vi "DCS.vi"(3 "error in":errorcluster) -> (10 "error out":errorcluster)   [LabVIEW 2013]
uses:
  <vilib>/Utility/miscctls.llb/LVPointTypeDef.ctl
  <vilib>/gmath/NumericalOptimization/Nonlinear Curve Fit LM.vi
  <userlib>/Accelerator/User Interface/Controls/dcs points.ctl
  <userlib>/Accelerator/User Interface/Controls/dcs_spot.ctl
  <vilib>/gmath/NI_Gmath.lvlib
panel:
  in  "Points to Check Noise":i32=2000
  in  "Color bar Control":cluster{dbl, u32}[](array[cluster])
  in  "stop":bool
  in  "Tab Control":T1(tab)
  out "Intensity Graph":dbl[][](graph)
  in  "Spot Save Folder":path=path "C:/Users/Clavius/Desktop/Spot Images"
  in  "Save Spot Image":bool
  in  "Clear Spot/Track":bool
  in  "Particle Limit":i64=500 min=0 step=10
  out "Laser spot\nMove (mm)":dbl[](array[numeric])=[nan, nan] format="%#.3g"
  out "Avg. Freq. (Hz)":dbl
  in  "Orange Cursor Position":dbl[](array[numeric])=[0.0, 0.0] min=-12.0 max=12.0 step=0.1 format="%.3g"
  out "Spot Widths":dbl[](array[numeric]) format="%.6g"
  out "Countdown to\nnext track point":i32=1
  out "XY Graph":cluster{"Y":dbl[], "Y":dbl[]}[](graph)
  in  "Load old position\nto Orange Cursor":bool
  in  "Set Orange Cursor\nto current position":bool
  out "# of Particles\nin Spot":dbl
  out "Current Spot Pos":dbl[](array[numeric])=[nan, nan] format="%.3g"
  in  "# of shots to calculate spot":i32=20
  out "Spot Size over time":dbl[][](graph)
  out "Filtered Signals":dbl[][](graph)
  out "Unfiltered Signals":ext[][](graph)
  in  "Auto Threshold":bool
  out "Sampling Frequency":u16(ring) items=["40 MHz", "20 MHz", "10 MHz", "5 MHz", "2.5 MHz", "1 MHz", "100 kHz", "10 kHz"]
  out "Length of Sample":dbl caption="s" format="%^#_3g"
  out "Memory Address Pointer":ext
  out "Post trigger Size":ext
  out "Pretrigger Size":ext
  out "Trigger Generation register":i32=23 format="%.0b"
  out "status register":i8=4 format="%08b"
  out "control register":i16=23 format="%015b"
  in  "Posttrigger size":i32
  in  "Acquisition Rate":u16(ring) items=["40 MHz", "20 MHz", "10 MHz", "5 MHz", "2.5 MHz", "1 MHz", "100 kHz", "10 kHz"]
  in  "Pretrigger size":i32=1000
  in  "Rising or falling?":bool
  out "Running Errors":errorcluster
  in  "Jorger TR slot":i32=3
  in  "Channels":i32[](array[numeric])=[0, 1, 2, 3, 4, 5, 6, 7]
  in  "Median Filter Rank":i32=30
  in  "Thresholds":ext[](array[numeric])
  in  "Level Buffer":i32=25
  in  "y":bool
  out "output":i32
  # "DAQ Parameter Indicators"
  # "DAQ Parameter Controls"
  # "Falling"
  # "Rising"
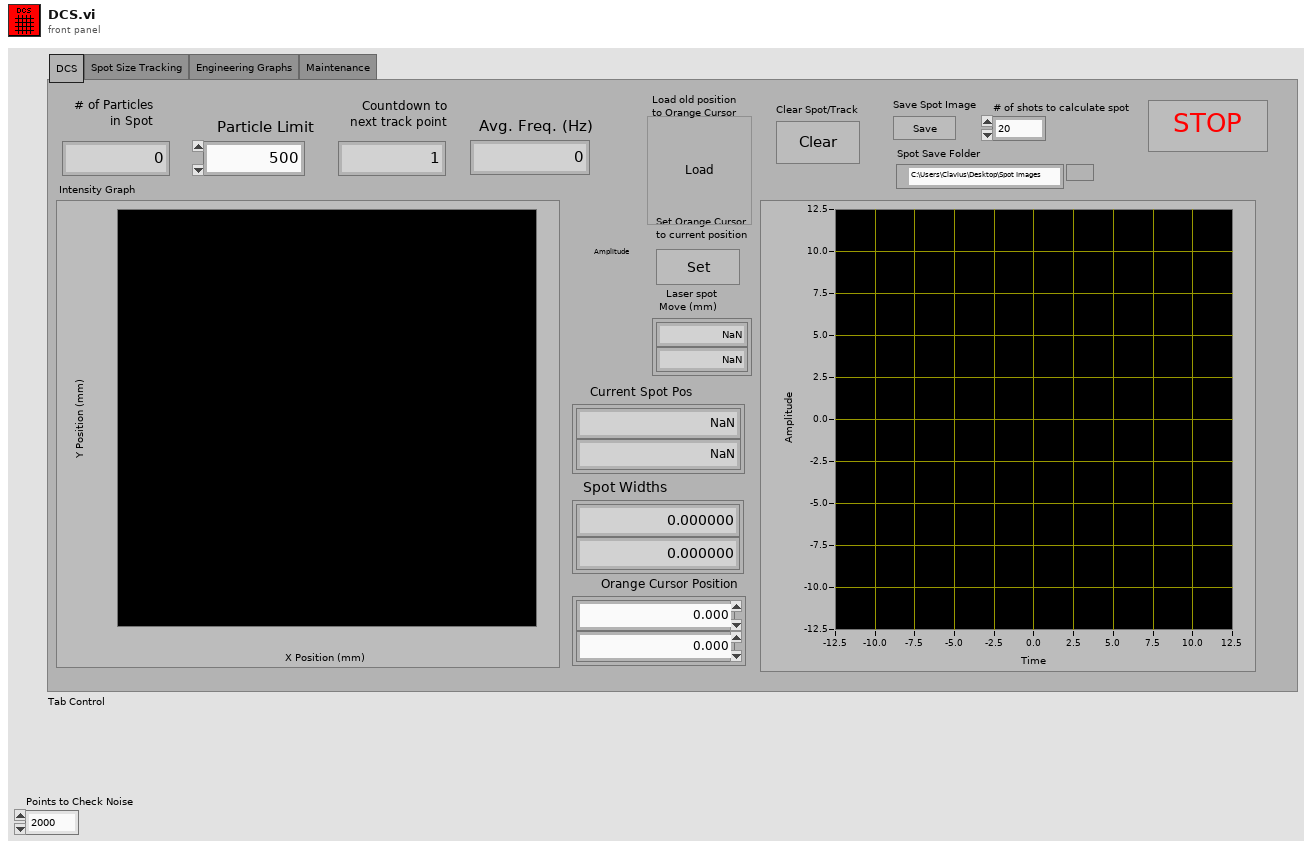
[diagram p1: front panel]
types:
  T1 = enum32{"DCS", "Spot Size Tracking", "Engineering Graphs", "Maintenance"}
  T2 = typedef "LVPointTypeDef.ctl" = cluster{"Horizontal":i16, "Vertical":i16}
  T3 = typedef "dcs_spot.ctl" = cluster{"DCS spot ID":i32, "Integer Timestamp":i64, "Spot X":dbl, "Spot Y":dbl, "Spot Width X":dbl, "Spot Width Y":dbl, "Spot Size":i32, "Experiment Settings ID":i32}
  T4 = typedef "dcs points.ctl" = cluster{"Integer Timestamp":i64, "X":dbl, "Y":dbl, "DCS spot ID":i32}
  T5 = typedef "imagedata.ctl" = cluster{"image type":i32, "image depth":i32, "image":u8[], "mask":u8[], "colors":u32[], "Rectangle":cluster{"left":i16, "top":i16, "right":i16, "bottom":i16}}
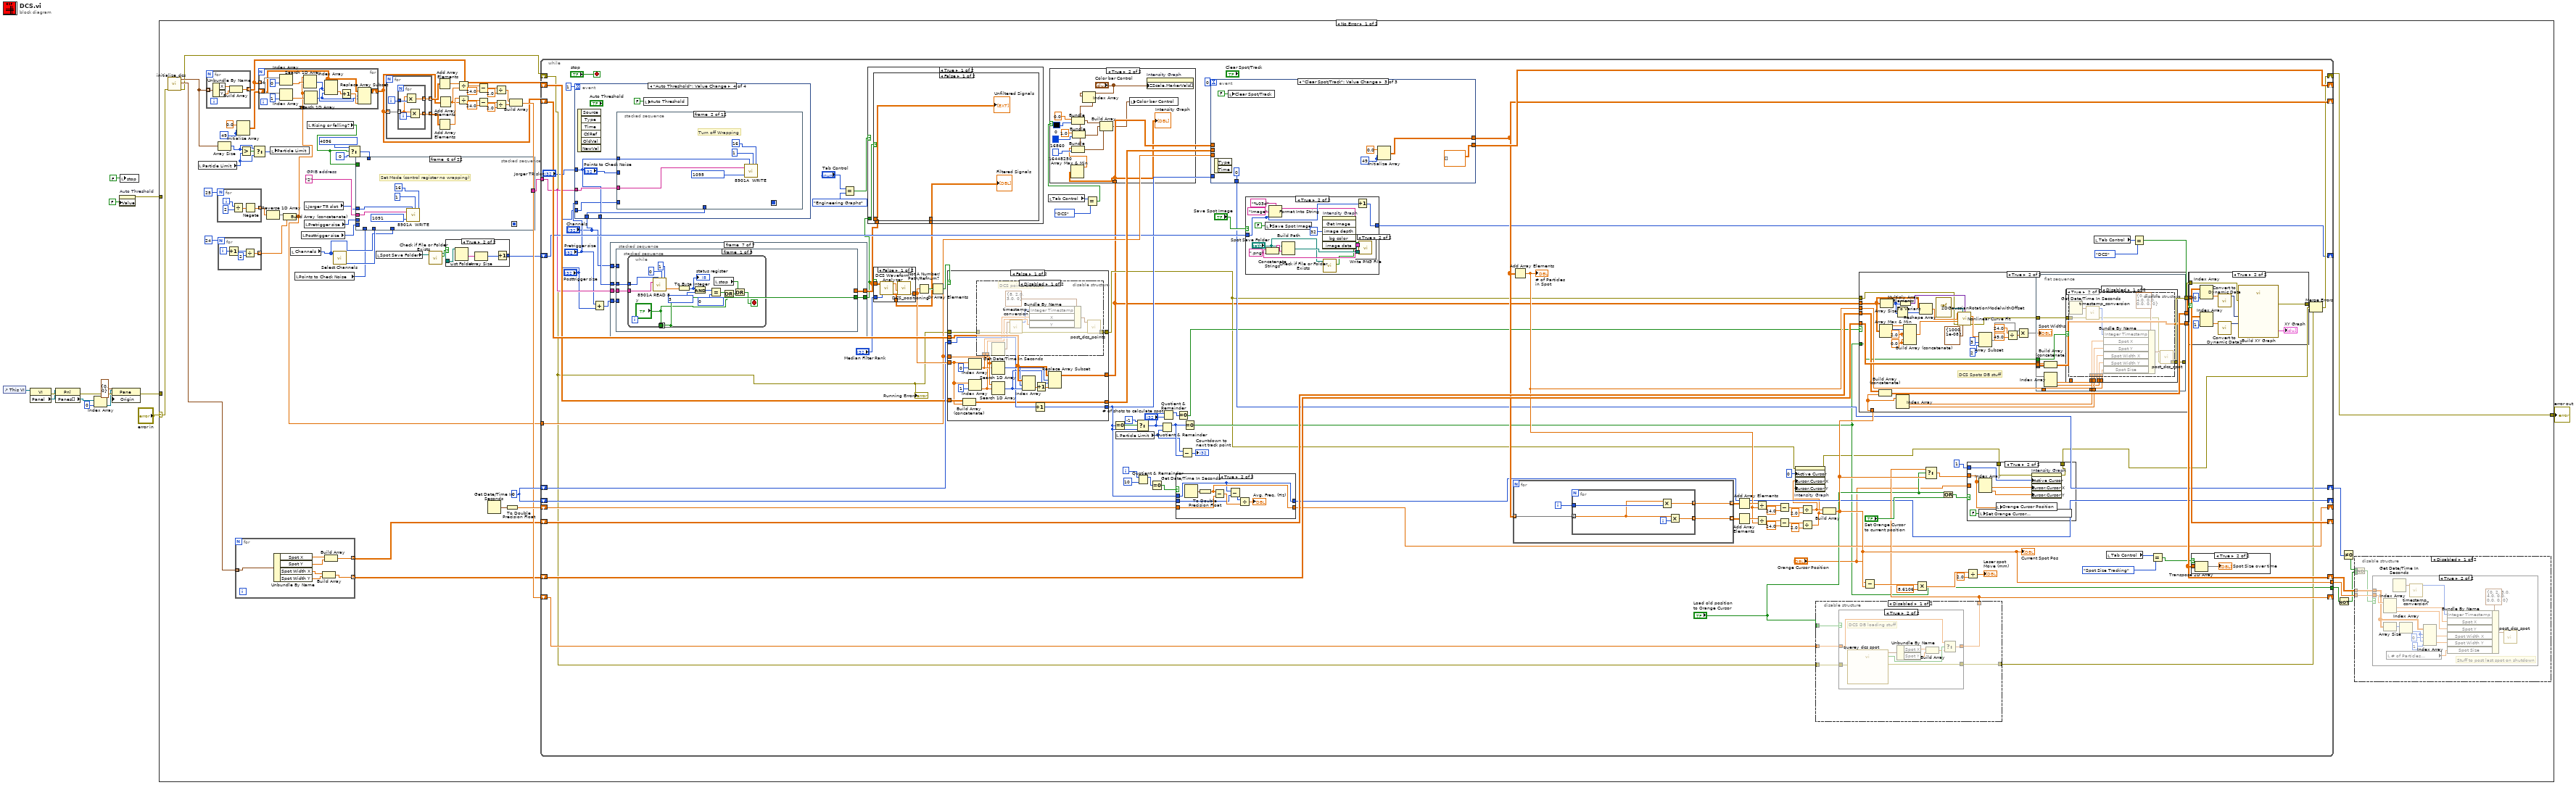
[diagram p0: block diagram]
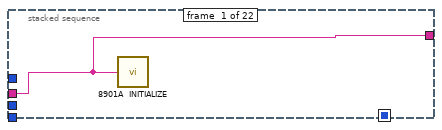
[diagram p4: hidden frame]
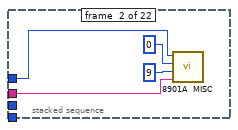
[diagram p5: hidden frame]
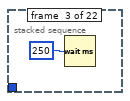
[diagram p6: hidden frame]
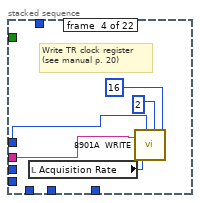
[diagram p7: hidden frame]
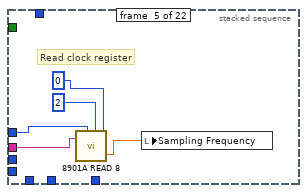
[diagram p8: hidden frame]
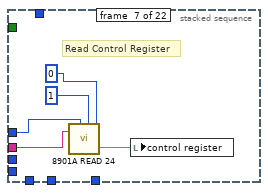
[diagram p9: hidden frame]
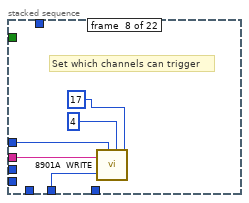
[diagram p10: hidden frame]
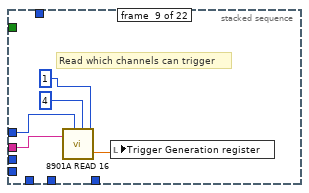
[diagram p11: hidden frame]
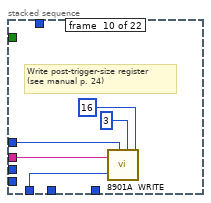
[diagram p12: hidden frame]
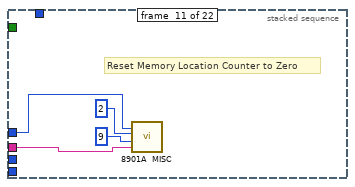
[diagram p13: hidden frame]
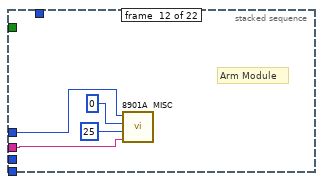
[diagram p14: hidden frame]
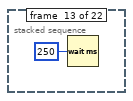
[diagram p15: hidden frame]
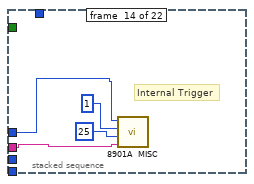
[diagram p16: hidden frame]
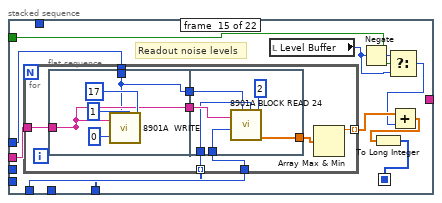
[diagram p17: hidden frame]
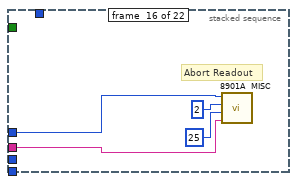
[diagram p18: hidden frame]
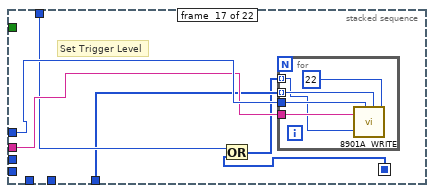
[diagram p19: hidden frame]
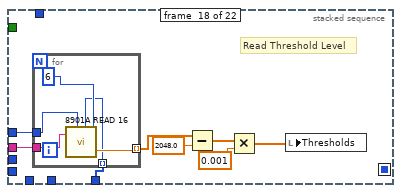
[diagram p20: hidden frame]
diagram:
  n1 = control-ref of="This VI"() -> (w11:refnum<vi>)
  n2 = property class="VI"(reference=w11) -> (error out=w10:errorcluster, "Panel"=w9:refnum<vi>)  [unwired: 1 in, 1 out]
  n3 = property class="Pnl"(reference=w9, error in=w10) -> (error out=w8:errorcluster, "Panes[]"=w7:refnum<vi>[])  [unwired: 1 out]
  n4 = Index Array(array=w7, index=0) -> (element=w5:refnum<vi>)
  n5 = property class="Pane"(reference=w5, error in=w8, "Origin"=T2 {"Horizontal"=0, "Vertical"=0}) -> (error out=w3:errorcluster)  [unwired: 1 out]
  n6 = property on="Auto Threshold" class="Bool (strict)"("Value"=FALSE ("Auto Threshold")) -> (error out=w1:errorcluster)  [unwired: 2 in, 1 out]
  n7 = local write "stop"(FALSE ("stop")) -> ()
  n8 = case shown="No Error" "error in" {
    selector: "error in" -> [w33 w956]
    tunnel: [w32 w956] -> w13
    tunnel: w3 -> [_ _]
    tunnel: w1 -> [_ _]
    frame No Error {
      w26 = "2"  # GPIB address
      w52 = 49 ("dimension size")
      w55 = 0
      n9 = call <userlib>:"initialize_dcs.vi"("error in (no error)"=w33) -> ("error out"=w27:errorcluster, "Dust Spot Array"=w44:T3[], "Dust Point Array"=w38:T4[])  [unwired: 8 in]
      n10 = local read "Particle Limit"() -> (w35:i64)
      n11 = for {
        tunnel: [w255] -> w43 mode=indexing
        tunnel: w38 -> [w254] mode=indexing
        n12 = Unbundle By Name(w254) -> ("X"=w257:dbl, "Y"=w256:dbl)
        n13 = Build Array(w257, w256) -> (w255:dbl[])
      }
      n14 = for {
        N: 25 -> [_]
        tunnel: [w271] -> w75 mode=indexing
        i -> [w274]
        n15 = Divide(x=w274, y=2) -> (x/y=w272:dbl)
        n16 = Negate(x=w272) -> (-x=w271:dbl)
      }
      n17 = Array Size(array=w38) -> (size(s)=w36:i32)
      n18 = for {
        N: 24 -> [_]
        tunnel: [w268] -> w73 mode=indexing
        i -> [w270]
        n19 = Increment(x=w270) -> (x+1=w267:i32)
        n20 = Divide(x=w267, y=2) -> (x/y=w268:dbl)
      }
      n21 = for {
        tunnel: [w249] -> w47 mode=indexing
        tunnel: [w248] -> w48 mode=indexing
        tunnel: w44 -> [w247] mode=indexing
        n22 = Unbundle By Name(w247) -> ("Spot X"=w253:dbl, "Spot Y"=w252:dbl, "Spot Width X"=w251:dbl, "Spot Width Y"=w250:dbl)
        n23 = Build Array(w251, w250) -> (w249:dbl[])
        n24 = Build Array(w253, w252) -> (w248:dbl[])
      }
      n25 = Initialize Array(0.0 ("element"), w52, w52) -> (w51:dbl[][])
      n26 = Greater?(x=w36, y=w35) -> (0:w37:bool)
      n27 = Select(t=w36, s=w37, f=w35) -> (s? t:f=w34:i64)
      n28 = Reverse 1D Array(array=w75) -> (reversed array=w74:dbl[])
      n29 = local write "Particle Limit"(w34) -> ()
      n30 = Build Array (concatenate)(w74, w73) -> (w49:dbl[])
      n31 = for {
        tunnel: w43 -> [w244] mode=indexing
        tunnel: w49 -> [w235]
        shift-right: [w236] -> w42
        shift-left: w51 -> [w237]
        n32 = Index Array(array=w244, index=0) -> (element=w243:dbl)
        n33 = Index Array(array=w244, index=1) -> (element=w242:dbl)
        n34 = Search 1D Array(1D array=w235, element=w243) -> (index of element=w239:i32)  [unwired: 1 in]
        n35 = Search 1D Array(1D array=w235, element=w242) -> (index of element=w238:i32)  [unwired: 1 in]
        n36 = Index Array(array=w237, index (row)=w239, index (col)=w238) -> (element=w241:dbl)
        n37 = Increment(x=w241) -> (x+1=w240:dbl)
        n38 = Replace Array Subset(array=w237, new element=w240, index (row)=w239, index (col)=w238) -> (w236:dbl[][])
      }
      n39 = local read "Channels"() -> (w17:i32[])
      n40 = local read "Points to Check Noise"() -> (w16:i32)
      n41 = local read "Posttrigger size"() -> (w22:i32)
      n42 = local read "Jorger TR slot"() -> (w24:i32)
      n43 = local read "Pretrigger size"() -> (w23:i32)
      n44 = local read "Rising or falling?"() -> (w15:bool)
      n45 = call <userlib>:"Select Channels.vi"("Channels"=w17) -> ("Channels in Use"=w21:u32)  [unwired: 10 in]
      n46 = Select(t=4096, s=w15, f=0) -> (s? t:f=w18:i32)
      n47 = stacked-sequence {
        seq-local: [_ _ _ _ _ _ _ _ _ _ _ _ _ _ w156 _ _ _ _ _ _ _] -> [_ _ _ _ _ _ _ _ _ _ _ _ _ _ _ _ w186 _ _ _ _ _]
        tunnel: w24 -> [_ w99 _ w106 w111 w114 w121 w125 w130 w136 w140 w143 _ w148 w158 w183 w191 w204 w212 w217 w222 w227]
        tunnel: w26 -> [w98 w100 _ w105 w110 w115 w120 w126 w131 w135 w139 w144 _ w149 w162 w182 w190 w203 w211 w216 w221 w226]
        tunnel: w23 -> [_ _ _ _ _ _ _ _ _ _ _ _ _ _ _ _ _ _ _ _ w220 _]
        tunnel: w22 -> [_ _ _ _ _ _ _ _ _ _ _ _ _ _ _ _ _ _ w210 _ _ _]
        tunnel: [w98 _ _ _ _ _ _ _ _ _ _ _ _ _ _ _ _ _ _ _ _ _] -> w25
        tunnel: w21 -> [_ _ _ _ _ _ _ w124 _ _ _ _ _ _ _ _ _ _ _ _ _ _]
        tunnel: w16 -> [_ _ _ _ _ _ _ _ _ w134 _ _ _ _ w161 _ _ _ _ _ _ _]
        tunnel: w18 -> [_ _ _ _ _ _ _ _ _ _ _ _ _ _ _ _ w189 _ _ _ _ _]
        tunnel: w17 -> [_ _ _ _ _ _ _ _ _ _ _ _ _ _ w159 _ w188 w198 _ _ _ _]
        tunnel: w15 -> [_ _ _ _ _ _ _ _ _ _ _ _ _ _ w153 _ _ _ _ _ _ _]
        frame #0 {
          n48 = call <instrlib>:"8901A  INITIALIZE.vi"("GPIB address"=w98) -> ()
        }
        frame #1 {
          n49 = call <instrlib>:"8901A  MISC.vi"("GPIB address"=w100, "f"=9, "a"=0, "n"=w99) -> ()
        }
        frame #2 {
          n50 = Wait (ms)(milliseconds to wait=250) -> ()  [unwired: 1 out]
        }
        frame #3 {
          # "Write TR clock register\n(see manual p. 20)"
          n51 = local read "Acquisition Rate"() -> (w104:u16)
          n52 = call <instrlib>:"8901A  WRITE.vi"("data"=w104, "GPIB address"=w105, "n"=w106, "a"=2, "f"=16) -> ()  [unwired: 1 in]
        }
        frame #4 {
          # "Read clock register"
          n53 = call <instrlib>:"8901A READ 8.vi"("GPIB address"=w110, "n"=w111, "a"=2, "f"=0) -> ("output"=w109:ext)  [unwired: 3 in]
          n54 = local write "Sampling Frequency"(w109) -> ()
        }
        frame #5 {
          # "Set Mode (control register no wrapping)"
          n55 = call <instrlib>:"8901A  WRITE.vi"("data"=1091, "GPIB address"=w115, "n"=w114, "a"=1, "f"=16) -> ()  [unwired: 1 in]
        }
        frame #6 {
          # "Read Control Register"
          n56 = call <instrlib>:"8901A READ 24.vi"("GPIB address"=w120, "n"=w121, "a"=1, "f"=0) -> ("output"=w119:ext)  [unwired: 3 in]
          n57 = local write "control register"(w119) -> ()
        }
        frame #7 {
          # "Set which channels can trigger"
          n58 = call <instrlib>:"8901A  WRITE.vi"("data"=w124, "GPIB address"=w126, "n"=w125, "a"=4, "f"=17) -> ()  [unwired: 1 in]
        }
        frame #8 {
          # "Read which channels can trigger"
          n59 = call <instrlib>:"8901A READ 16.vi"("GPIB address"=w131, "n"=w130, "a"=u8 4, "f"=u8 1) -> ("output"=w129:ext)  [unwired: 3 in]
          n60 = local write "Trigger Generation register"(w129) -> ()
        }
        frame #9 {
          # "Write post-trigger-size register\n(see manual p. 24)"
          n61 = call <instrlib>:"8901A  WRITE.vi"("data"=w134, "GPIB address"=w135, "n"=w136, "a"=3, "f"=16) -> ()  [unwired: 1 in]
        }
        frame #10 {
          # "Reset Memory Location Counter to Zero"
          n62 = call <instrlib>:"8901A  MISC.vi"("GPIB address"=w139, "f"=u8 9, "a"=u8 2, "n"=w140) -> ()
        }
        frame #11 {
          # "Arm Module"
          n63 = call <instrlib>:"8901A  MISC.vi"("GPIB address"=w144, "f"=25, "a"=0, "n"=w143) -> ()
        }
        frame #12 {
          n64 = Wait (ms)(milliseconds to wait=u32 250) -> ()  [unwired: 1 out]
        }
        frame #13 {
          # "Internal Trigger"
          n65 = call <instrlib>:"8901A  MISC.vi"("GPIB address"=w149, "f"=u8 25, "a"=u8 1, "n"=w148) -> ()
        }
        frame #14 {
          # "Readout noise levels"
          n66 = for {
            tunnel: w162 -> [w169]
            tunnel: w161 -> [w168]
            tunnel: [w166] -> w160 mode=indexing
            tunnel: w159 -> [w165] mode=indexing
            tunnel: w158 -> [w164]
            n67 = flat-sequence {
              tunnel: [w173] -> _
              tunnel: [w173] -> w170
              tunnel: w169 -> [w173]
              tunnel: w164 -> [w171]
              tunnel: [w171] -> w163
              tunnel: w170 -> [w180]
              tunnel: [w179] -> w167
              tunnel: w168 -> [w178]
              tunnel: w165 -> [w177]
              tunnel: w163 -> [w176]
              frame #0 {
                n68 = call <instrlib>:"8901A  WRITE.vi"("data"=0, "GPIB address"=w173, "n"=w171, "a"=1, "f"=17) -> ()  [unwired: 1 in]
              }
              frame #1 {
                n69 = call <instrlib>:"8901A BLOCK READ 24.vi"("f"=2, "a"=w177, "n"=w176, "GPIB address"=w180, "# points to read"=w178) -> ("output"=w179:ext[])  [unwired: 4 in]
              }
            }
            n70 = Array Max & Min(array=w167) -> (max value=w166:ext)  [unwired: 3 out]
          }
          n71 = local read "Level Buffer"() -> (w155:i32)
          n72 = Negate(x=w155) -> (-x=w154:i32)
          n73 = Select(t=w154, s=w153, f=w155) -> (s? t:f=w152:i32)
          n74 = Add(x=w160, y=w152) -> (x+y=w157:ext[])
          n75 = To Long Integer(number=w157) -> (32bit integer=w156:i32[])
        }
        frame #15 {
          # "Abort Readout"
          n76 = call <instrlib>:"8901A  MISC.vi"("GPIB address"=w182, "f"=25, "a"=2, "n"=w183) -> ()
        }
        frame #16 {
          # "Set Trigger Level"
          n77 = Or(x=w189, y=w186) -> (x .or. y?=w187:i32[])
          n78 = for {
            tunnel: w191 -> [w195]
            tunnel: w190 -> [w194]
            tunnel: w188 -> [w193] mode=indexing
            tunnel: w187 -> [w192] mode=indexing
            n79 = call <instrlib>:"8901A  WRITE.vi"("data"=w192, "GPIB address"=w194, "n"=w195, "a"=w193, "f"=u8 22) -> ()  [unwired: 1 in]
          }
        }
        frame #17 {
          # "Read Threshold Level"
          n80 = for {
            tunnel: w204 -> [w208]
            tunnel: w203 -> [w207]
            tunnel: [w206] -> w201 mode=indexing
            tunnel: w198 -> [w205] mode=indexing
            n81 = call <instrlib>:"8901A READ 16.vi"("GPIB address"=w207, "n"=w208, "a"=w205, "f"=u8 6) -> ("output"=w206:ext)  [unwired: 3 in]
          }
          n82 = Subtract(x=w201, y=2048.0) -> (x-y=w199:ext[])
          n83 = Multiply(x=w199, y=0.001) -> (x*y=w197:ext[])
          n84 = local write "Thresholds"(w197) -> ()
        }
        frame #18 {
          # "Write post-trigger-size register\n(see manual p. 24)"
          n85 = call <instrlib>:"8901A  WRITE.vi"("data"=w210, "GPIB address"=w211, "n"=w212, "a"=3, "f"=16) -> ()  [unwired: 1 in]
        }
        frame #19 {
          # "Read Post trigger size"
          n86 = call <instrlib>:"8901A READ 24.vi"("GPIB address"=w216, "n"=w217, "a"=3, "f"=0) -> ("output"=w215:ext)  [unwired: 3 in]
          n87 = local write "Post trigger Size"(w215) -> ()
        }
        frame #20 {
          # "Write Pretrigger size"
          n88 = call <instrlib>:"8901A  WRITE.vi"("data"=w220, "GPIB address"=w221, "n"=w222, "a"=4, "f"=16) -> ()  [unwired: 1 in]
        }
        frame #21 {
          # "Read Pretrigger size"
          n89 = call <instrlib>:"8901A READ 16.vi"("GPIB address"=w226, "n"=w227, "a"=u8 4, "f"=u8 0) -> ("output"=w225:ext)  [unwired: 3 in]
          n90 = local write "Pretrigger Size"(w225) -> ()
        }
      }
      n91 = local read "Spot Save Folder"() -> (w30:path)
      n92 = for {
        tunnel: w42 -> [w261] mode=indexing
        tunnel: [w259] -> w72 mode=indexing
        tunnel: [w258] -> w71 mode=indexing
        i -> [w260]
        n93 = for {
          tunnel: w261 -> [w263] mode=indexing
          tunnel: w260 -> [w266]
          tunnel: [w264] -> w258 mode=indexing
          tunnel: [w262] -> w259 mode=indexing
          i -> [w265]
          n94 = Multiply(x=w263, y=w266) -> (x*y=w262:dbl)
          n95 = Multiply(x=w263, y=w265) -> (x*y=w264:dbl)
        }
      }
      n96 = call <vilib>:"Check if File or Folder Exists.vi"("path"=w30) -> ("file or folder exists?"=w29:bool, "dup path"=w28:path)  [unwired: 8 in, 1 out]
      n97 = Add Array Elements(numeric array=w72) -> (sum=w70:dbl)
      n98 = Add Array Elements(numeric array=w71) -> (sum=w69:dbl)
      n99 = Add Array Elements(numeric array=w42) -> (sum=w61:dbl)
      n100 = case shown="True" w29 {
        tunnel: [0 w232] -> w31
        tunnel: w28 -> [_ w231]
        frame False {
        }
        frame True {
          n101 = List Folder(path=w231) -> (filenames=w234:string[])  [unwired: 3 in, 3 out]
          n102 = Array Size(array=w234) -> (size(s)=w233:i32)
          n103 = Increment(x=w233) -> (x+1=w232:i32)
        }
      }
      n104 = Divide(x=w70, y=w61) -> (x/y=w68:dbl)
      n105 = Divide(x=w69, y=w61) -> (x/y=w67:dbl)
      n106 = Subtract(x=w68, y=24.0) -> (x-y=w59:dbl)
      n107 = Subtract(x=w67, y=24.0) -> (x-y=w65:dbl)
      n108 = Get Date/Time In Seconds() -> (seconds since 1Jan1904=w57:timestamp)
      n109 = Divide(x=w59, y=2.0) -> (x/y=w58:dbl)
      n110 = Divide(x=w65, y=2.0) -> (x/y=w62:dbl)
      n111 = To Double Precision Float(number=w57) -> (double precision float=w56:dbl)
      n112 = Build Array(w58, w62) -> (w50:dbl[])
      n113 = while {
        shift-right: [w351] -> _
        shift-left: w43 -> [w353]
        shift-right: [w336] -> _
        shift-left: w42 -> [w376]
        tunnel: w49 -> [w327]
        shift-right: [w335] -> _
        shift-left: w50 -> [w364]
        tunnel: [w350] -> w54
        shift-right: [w326] -> w32
        shift-left: w27 -> [w281]
        shift-right: [w348] -> _
        shift-left: w48 -> [w340]
        shift-right: [w317] -> w41
        shift-left: w55 -> [w354]
        shift-right: [w349] -> w45
        shift-left: w47 -> [w352]
        shift-right: [w333] -> _
        shift-left: w56 -> [w347]
        shift-right: [w332] -> _
        shift-left: w55 -> [w334]
        tunnel: [w314] -> w46
        shift-right: [w319] -> _
        shift-left: w31 -> [w320]
        tunnel: w25 -> [w286]
        i -> [w297]
        stop <- "stop" stop-if-true
        n114 = event shown="[3] \"Auto Threshold\": Value Change" {
          selector: _ -> [_ _ _ _]
          dyn-events: _ -> [_ _ _ _]
          timeout: 1 -> [_ _ _ _]
          tunnel: w286 -> [_ w516 w581 w617]
          tunnel: "Pretrigger size" -> [_ w515 _ _]
          tunnel: "Posttrigger size" -> [_ w514 _ w612]
          tunnel: [w503 w504 w580 w614] -> w285
          tunnel: "Channels" -> [_ w506 w579 w615]
          tunnel: "Jorger TR slot" -> [_ w504 w580 w614]
          event Timeout {
            n115 = event-data() -> ()  [unwired: 1 in, 3 out]
            n116 = local read "Jorger TR slot"() -> (w503:i32)
          }
          event "Acquisition Rate", "Pretrigger size", "Posttrigger size": Value Change {
            n117 = event-data() -> ()  [unwired: 1 in, 6 out]
            n118 = local read "Acquisition Rate"() -> (w513:u16)
            n119 = call <userlib>:"Select Channels.vi"("Channels"=w506) -> ("Channels in Use"=w505:u32)  [unwired: 10 in]
            n120 = stacked-sequence {
              tunnel: w504 -> [w551 w556 w561 w566 w571 w576]
              tunnel: w516 -> [w550 w555 w560 w565 w570 w575]
              tunnel: w515 -> [_ _ _ _ w569 _]
              tunnel: w514 -> [w549 _ _ _ _ _]
              tunnel: w505 -> [_ _ _ _ _ _]
              frame #0 {
                # "Write post-trigger-size register\n(see manual p. 24)"
                n121 = call <instrlib>:"8901A  WRITE.vi"("data"=w549, "GPIB address"=w550, "n"=w551, "a"=3, "f"=16) -> ()  [unwired: 1 in]
              }
              frame #1 {
                # "Read Post trigger size"
                n122 = call <instrlib>:"8901A READ 24.vi"("GPIB address"=w555, "n"=w556, "a"=3, "f"=0) -> ("output"=→"Post trigger Size":ext)  [unwired: 3 in]
              }
              frame #2 {
                # "Write TR clock register\n(see manual p. 20)"
                n123 = call <instrlib>:"8901A  WRITE.vi"("data"="Acquisition Rate", "GPIB address"=w560, "n"=w561, "a"=2, "f"=16) -> ()  [unwired: 1 in]
              }
              frame #3 {
                # "Read clock register"
                n124 = call <instrlib>:"8901A READ 8.vi"("GPIB address"=w565, "n"=w566, "a"=2, "f"=0) -> ("output"=→"Sampling Frequency":ext)  [unwired: 3 in]
              }
              frame #4 {
                # "Write Pretrigger size"
                n125 = call <instrlib>:"8901A  WRITE.vi"("data"=w569, "GPIB address"=w570, "n"=w571, "a"=4, "f"=16) -> ()  [unwired: 1 in]
              }
              frame #5 {
                # "Read Pretrigger size"
                n126 = call <instrlib>:"8901A READ 16.vi"("GPIB address"=w575, "n"=w576, "a"=u8 4, "f"=u8 0) -> ("output"=→"Pretrigger Size":ext)  [unwired: 3 in]
              }
            }
            n127 = case shown="0, Default" w513 {
              tunnel: [w517 w521 w525 w529 w533 w537 w541 w545] -> w511
              frame 0, Default {
                n128 = Power Of 10(x=6) -> (10^x=w519:dbl)
                n129 = Multiply(x=40, y=w519) -> (x*y=w517:dbl)
              }
              frame 1 {
                n130 = Power Of 10(x=6) -> (10^x=w523:dbl)
                n131 = Multiply(x=20, y=w523) -> (x*y=w521:dbl)
              }
              frame 2 {
                n132 = Power Of 10(x=6) -> (10^x=w527:dbl)
                n133 = Multiply(x=10, y=w527) -> (x*y=w525:dbl)
              }
              frame 3 {
                n134 = Power Of 10(x=6) -> (10^x=w531:dbl)
                n135 = Multiply(x=5, y=w531) -> (x*y=w529:dbl)
              }
              frame 4 {
                n136 = Power Of 10(x=6) -> (10^x=w535:dbl)
                n137 = Multiply(x=2.5, y=w535) -> (x*y=w533:dbl)
              }
              frame 5 {
                n138 = Power Of 10(x=6) -> (10^x=w539:dbl)
                n139 = Multiply(x=1, y=w539) -> (x*y=w537:dbl)
              }
              frame 6 {
                n140 = Power Of 10(x=3) -> (10^x=w543:dbl)
                n141 = Multiply(x=100, y=w543) -> (x*y=w541:dbl)
              }
              frame 7 {
                n142 = Power Of 10(x=3) -> (10^x=w547:dbl)
                n143 = Multiply(x=10, y=w547) -> (x*y=w545:dbl)
              }
            }
            n144 = local read "Posttrigger size"() -> (w510:i32)
            n145 = Reciprocal(x=w511) -> (1/x=w512:dbl)
            n146 = local read "Pretrigger size"() -> (w509:i32)
            n147 = Add(x=w510, y=w509) -> (x+y=w508:i32)
            n148 = Multiply(x=w508, y=w512) -> (x*y=→"Length of Sample":dbl)
          }
          event "Channels", "Thresholds", "Rising or falling?": Value Change {
            n149 = event-data() -> ()  [unwired: 1 in, 6 out]
            n150 = stacked-sequence {
              tunnel: w581 -> [w585 w589 w597]
              tunnel: w580 -> [w584 w590 w596]
              tunnel: w579 -> [w582 _ w595]
              frame #0 {
                n151 = call <userlib>:"Select Channels.vi"("Channels"=w582) -> ("Channels in Use"=w583:u32)  [unwired: 10 in]
                n152 = call <instrlib>:"8901A  WRITE.vi"("data"=w583, "GPIB address"=w585, "n"=w584, "a"=4, "f"=17) -> ()  [unwired: 1 in]
              }
              frame #1 {
                n153 = call <instrlib>:"8901A READ 16.vi"("GPIB address"=w589, "n"=w590, "a"=u8 4, "f"=u8 1) -> ("output"=→"Trigger Generation register":ext)  [unwired: 3 in]
              }
              frame #2 {
                n154 = Add(x="Thresholds", y=2.048) -> (x+y=w605:ext[])
                n155 = Multiply(x=w605, y=1000.0) -> (x*y=w603:ext[])
                n156 = Select(t=4096, s="Rising or falling?", f=0) -> (s? t:f=w599:i32)
                n157 = To Long Integer(number=w603) -> (32bit integer=w600:i32[])
                n158 = Or(x=w599, y=w600) -> (x .or. y?=w598:i32[])
                n159 = for {
                  tunnel: w596 -> [w610]
                  tunnel: w597 -> [w609]
                  tunnel: w595 -> [w608] mode=indexing
                  tunnel: w598 -> [w607] mode=indexing
                  n160 = call <instrlib>:"8901A  WRITE.vi"("data"=w607, "GPIB address"=w609, "n"=w610, "a"=w608, "f"=u8 22) -> ()  [unwired: 1 in]
                }
              }
            }
          }
          event "Auto Threshold": Value Change {
            n161 = event-data() -> ()  [unwired: 1 in, 6 out]
            n162 = stacked-sequence {
              seq-local: [_ _ _ _ _ _ _ w647 _ _ _ _] -> [_ _ _ _ _ _ _ _ _ w680 _ _]
              tunnel: w617 -> [w620 w624 w628 w632 w636 _ w641 w651 w675 w682 w695 w708]
              tunnel: "Points to Check Noise" -> [w619 _ _ _ _ _ _ w649 _ _ _ _]
              tunnel: w614 -> [w618 w623 w629 w633 w637 _ w642 w650 w676 w681 w694 w707]
              tunnel: w615 -> [_ _ _ _ _ _ _ w648 _ w683 w696 _]
              tunnel: w612 -> [_ _ _ _ _ _ _ _ _ _ _ w706]
              frame #0 {
                # "Write post-trigger-size register\n(see manual p. 24)"
                n163 = call <instrlib>:"8901A  WRITE.vi"("data"=w619, "GPIB address"=w620, "n"=w618, "a"=3, "f"=16) -> ()  [unwired: 1 in]
              }
              frame #1 {
                # "Turn off Wrapping"
                n164 = call <instrlib>:"8901A  WRITE.vi"("data"=1095, "GPIB address"=w624, "n"=w623, "a"=1, "f"=16) -> ()  [unwired: 1 in]
              }
              frame #2 {
                # "Reset Memory Counter to Zero"
                n165 = call <instrlib>:"8901A  MISC.vi"("GPIB address"=w628, "f"=u8 9, "a"=u8 2, "n"=w629) -> ()
              }
              frame #3 {
                # "Arm Module"
                n166 = call <instrlib>:"8901A  MISC.vi"("GPIB address"=w632, "f"=25, "a"=0, "n"=w633) -> ()
              }
              frame #4 {
                n167 = call <instrlib>:"8901A  MISC.vi"("GPIB address"=w636, "f"=u8 21, "a"=u8 2, "n"=w637) -> ()
              }
              frame #5 {
                n168 = Wait (ms)(milliseconds to wait=u32 250) -> ()  [unwired: 1 out]
              }
              frame #6 {
                # "Internal Trigger"
                n169 = call <instrlib>:"8901A  MISC.vi"("GPIB address"=w641, "f"=u8 25, "a"=u8 1, "n"=w642) -> ()
              }
              frame #7 {
                n170 = for {
                  tunnel: w651 -> [w662]
                  tunnel: w649 -> [w661]
                  tunnel: [w659] -> w655 mode=indexing
                  tunnel: w648 -> [w658] mode=indexing
                  tunnel: w650 -> [w657]
                  n171 = flat-sequence {
                    tunnel: [w666] -> _
                    tunnel: [w666] -> w663
                    tunnel: w662 -> [w666]
                    tunnel: w657 -> [w664]
                    tunnel: [w664] -> w656
                    tunnel: w663 -> [w673]
                    tunnel: [w672] -> w660
                    tunnel: w661 -> [w671]
                    tunnel: w658 -> [w670]
                    tunnel: w656 -> [w669]
                    frame #0 {
                      n172 = call <instrlib>:"8901A  WRITE.vi"("data"=0, "GPIB address"=w666, "n"=w664, "a"=1, "f"=17) -> ()  [unwired: 1 in]
                    }
                    frame #1 {
                      n173 = call <instrlib>:"8901A BLOCK READ 24.vi"("f"=2, "a"=w670, "n"=w669, "GPIB address"=w673, "# points to read"=w671) -> ("output"=w672:ext[])  [unwired: 4 in]
                    }
                  }
                  n174 = Array Max & Min(array=w660) -> (max value=w659:ext)  [unwired: 3 out]
                }
                n175 = local read "Rising or falling?"() -> (w645:bool)
                n176 = Negate(x="Level Buffer") -> (-x=w653:i32)
                n177 = Select(t=w653, s=w645, f="Level Buffer") -> (s? t:f=w652:i32)
                n178 = Add(x=w655, y=w652) -> (x+y=w654:ext[])
                n179 = To Long Integer(number=w654) -> (32bit integer=w647:i32[])
              }
              frame #8 {
                # "Abort Readout"
                n180 = call <instrlib>:"8901A  MISC.vi"("GPIB address"=w675, "f"=25, "a"=2, "n"=w676) -> ()
              }
              frame #9 {
                n181 = local read "Rising or falling?"() -> (w679:bool)
                n182 = Select(t=4096, s=w679, f=0) -> (s? t:f=w684:i32)
                n183 = Or(x=w684, y=w680) -> (x .or. y?=w687:i32[])
                n184 = for {
                  tunnel: w681 -> [w691]
                  tunnel: w682 -> [w690]
                  tunnel: w683 -> [w689] mode=indexing
                  tunnel: w687 -> [w688] mode=indexing
                  n185 = call <instrlib>:"8901A  WRITE.vi"("data"=w688, "GPIB address"=w690, "n"=w691, "a"=w689, "f"=u8 22) -> ()  [unwired: 1 in]
                }
              }
              frame #10 {
                n186 = for {
                  tunnel: w694 -> [w704]
                  tunnel: w695 -> [w703]
                  tunnel: [w702] -> w697 mode=indexing
                  tunnel: w696 -> [w701] mode=indexing
                  n187 = call <instrlib>:"8901A READ 16.vi"("GPIB address"=w703, "n"=w704, "a"=w701, "f"=u8 6) -> ("output"=w702:ext)  [unwired: 3 in]
                }
                n188 = Subtract(x=w697, y=2048.0) -> (x-y=w698:ext[])
                n189 = Multiply(x=w698, y=0.001) -> (x*y=w693:ext[])
                n190 = local write "Thresholds"(w693) -> ()
              }
              frame #11 {
                # "Write post-trigger-size register\n(see manual p. 24)"
                n191 = call <instrlib>:"8901A  WRITE.vi"("data"=w706, "GPIB address"=w708, "n"=w707, "a"=3, "f"=16) -> ()  [unwired: 1 in]
              }
            }
            n192 = local write "Auto Threshold"(FALSE ("Auto Threshold")) -> ()
          }
        }
        n193 = Add(x="Pretrigger size", y="Posttrigger size") -> (x+y=w282:i32)
        n194 = stacked-sequence {
          tunnel: w285 -> [w402 w407 w411 w414 w420 w425 w433]
          tunnel: w286 -> [w401 w406 w410 w415 w421 w426 w434]
          tunnel: [_ _ _ _ _ _ w432] -> w277
          tunnel: w282 -> [_ _ _ _ _ _ w431]
          tunnel: "Channels" -> [_ _ _ _ _ _ w430]
          tunnel: [_ _ _ _ _ _ w429] -> w279
          frame #0 {
            # "Set Control Register"
            n195 = call <instrlib>:"8901A  WRITE.vi"("data"=1095, "GPIB address"=w401, "n"=w402, "a"=1, "f"=16) -> ()  [unwired: 1 in]
          }
          frame #1 {
            # "Read Control Register"
            n196 = call <instrlib>:"8901A READ 24.vi"("GPIB address"=w406, "n"=w407, "a"=1, "f"=0) -> ("output"=→"control register":ext)  [unwired: 3 in]
          }
          frame #2 {
            # "Reset Memory Location counter to 0"
            n197 = call <instrlib>:"8901A  MISC.vi"("GPIB address"=w410, "f"=u8 9, "a"=u8 2, "n"=w411) -> ()
          }
          frame #3 {
            n198 = disable-structure shown="Disabled" {
              disable-tunnel: w415 -> [w417 _]
              disable-tunnel: w414 -> [w416 _]
              frame Disabled {
                # "Clear All Valid Trigger tags"
                n199 = call <instrlib>:"8901A  MISC.vi"("GPIB address"=w417, "f"=u8 21, "a"=u8 2, "n"=w416) -> ()
              }
              frame Enabled {
              }
            }
          }
          frame #4 {
            # "Arm Module"
            n200 = call <instrlib>:"8901A  MISC.vi"("GPIB address"=w421, "f"=25, "a"=0, "n"=w420) -> ()
          }
          frame #5 {
            n201 = call <instrlib>:"8901A READ 8.vi"("GPIB address"=w426, "n"=w425, "a"=0, "f"=1) -> ("output"=→"output":ext)  [unwired: 3 in]
          }
          frame #6 {
            n202 = stacked-sequence {
              seq-local: [w435 _ _ _ _] -> [_ w454 w465 _ _]
              tunnel: w434 -> [w437 w452 w462 w494 w499]
              tunnel: w433 -> [w436 w453 w461 w495 w500]
              tunnel: [w435 _ _ _ _] -> w432
              tunnel: w431 -> [_ _ w464 _ _]
              tunnel: w430 -> [_ _ w463 _ _]
              tunnel: [_ _ w460 _ _] -> w429
              frame #0 {
                n203 = while {
                  tunnel: w437 -> [w444]
                  tunnel: w436 -> [w443]
                  tunnel: ["y"] -> w435
                  stop <- w442 stop-if-true
                  n204 = call <instrlib>:"8901A READ 8.vi"("GPIB address"=w444, "n"=w443, "a"=0, "f"=1) -> ("output"=w447:ext)  [unwired: 3 in]
                  n205 = To Byte Integer(number=w447) -> (8bit integer=w441:i8)
                  "status register" <- w441
                  n206 = And(x=w441, y=i8 3) -> (x .and. y?=w448:i8)
                  n207 = Equal?(x=w448, y=i8 0) -> (x = y?=w440:bool)
                  n208 = local read "stop"() -> (w439:bool)
                  n209 = Or(x=w440, y="y") -> (x .or. y?=w449:bool)
                  n210 = Or(x=w439, y=w449) -> (x .or. y?=w442:bool)
                }
              }
              frame #1 {
                n211 = case shown="False" w454 {
                  tunnel: w453 -> [w457 _]
                  tunnel: w452 -> [w456 _]
                  frame False {
                    n212 = call <instrlib>:"8901A READ 24.vi"("GPIB address"=w456, "n"=w457, "a"=u8 9, "f"=u8 0) -> ("output"=→"Memory Address Pointer":ext)  [unwired: 3 in]
                  }
                  frame True {
                  }
                }
              }
              frame #2 {
                n213 = case shown="True" w465 {
                  tunnel: w464 -> [_ w471]
                  tunnel: w463 -> [_ w472]
                  tunnel: w462 -> [_ w470]
                  tunnel: w461 -> [_ w469]
                  tunnel: [ext[][] [[nan]] ("output") w467] -> w460
                  frame False {
                  }
                  frame True {
                    n214 = local read "Memory Address Pointer"() -> (w468:ext)
                    n215 = for {
                      N: 8 -> [_]
                      tunnel: w472 -> [w476] mode=indexing
                      tunnel: w471 -> [w475]
                      tunnel: w470 -> [w480]
                      tunnel: w469 -> [w479]
                      tunnel: w468 -> [w482]
                      tunnel: [w474] -> w467 mode=indexing
                      n216 = Subtract(x=w482, y=w475) -> (x-y=w481:ext)
                      n217 = flat-sequence {
                        tunnel: w481 -> [w485]
                        tunnel: w480 -> [w483]
                        tunnel: w479 -> [w484]
                        tunnel: [w484] -> w478
                        tunnel: [w483] -> w477
                        tunnel: w478 -> [w491]
                        tunnel: w477 -> [w490]
                        tunnel: w476 -> [w492]
                        tunnel: w475 -> [w489]
                        tunnel: [w488] -> w474
                        frame #0 {
                          n218 = call <instrlib>:"8901A  WRITE.vi"("data"=w485, "GPIB address"=w483, "n"=w484, "a"=1, "f"=17) -> ()  [unwired: 1 in]
                        }
                        frame #1 {
                          n219 = call <instrlib>:"8901A BLOCK READ 24.vi"("f"=2, "a"=w492, "n"=w491, "GPIB address"=w490, "# points to read"=w489) -> ("output"=w488:ext[])  [unwired: 4 in]
                        }
                      }
                    }
                  }
                }
              }
              frame #3 {
                # "Abort Readout"
                n220 = call <instrlib>:"8901A  MISC.vi"("GPIB address"=w494, "f"=25, "a"=2, "n"=w495) -> ()
              }
              frame #4 {
                # "Read in control register"
                n221 = call <instrlib>:"8901A READ 24.vi"("GPIB address"=w499, "n"=w500, "a"=1, "f"=0) -> ("output"=w498:ext)  [unwired: 3 in]
                n222 = local write "control register"(w498) -> ()
              }
            }
          }
        }
        n223 = Equal?(x="Tab Control", y=T1."Engineering Graphs") -> (x = y?=w308:bool)
        n224 = case shown="False" w277 {
          tunnel: [w397 dbl[] [nan] ("X-Y position")] -> w361
          tunnel: w279 -> [w395 _]
          tunnel: "Median Filter Rank" -> [w394 _]
          tunnel: [w393 dbl[][] [] ("Filtered Signals")] -> w278
          frame False {
            n225 = call <userlib>:"DCS Waveform Analyzer.vi"("Rank"=w394, "8 DCS Waveforms"=w395) -> ("Filtered Signals"=w393:dbl[][], "Maxs"=w396:dbl[])  [unwired: 8 in]
            n226 = call <userlib>:"DCS_positioning.vi"("Data"=w396) -> ("X-Y position"=w397:dbl[])  [unwired: 10 in]
          }
          frame True {
          }
        }
        n227 = case shown="True" w308 {
          tunnel: w279 -> [w752 _]
          tunnel: w278 -> [w751 _]
          tunnel: w277 -> [w750 _]
          frame True {
            n228 = case shown="False" w750 {
              tunnel: w752 -> [w754 _]
              tunnel: w751 -> [w753 _]
              frame False {
                "Filtered Signals" <- w753
                "Unfiltered Signals" <- w754
              }
              frame True {
              }
            }
          }
          frame False {
          }
        }
        n229 = Not A Number/Path/Refnum?(number/path/refnum=w361) -> (NaN/Path/Refnum?=w375:bool[])
        n230 = Or Array Elements(Boolean array=w375) -> (logical OR=w360:bool)
        n231 = case shown="False" w360 {
          tunnel: w376 -> [w940 w955]
          tunnel: [w935 w955] -> w298
          tunnel: w327 -> [w934 _]
          tunnel: w361 -> [w930 _]
          tunnel: w354 -> [w933 w954]
          tunnel: [w932 w954] -> w318
          tunnel: w353 -> [w931 w953]
          tunnel: [w929 w953] -> w330
          tunnel: w281 -> [w926 w952]
          tunnel: [w925 w952] -> w303
          frame False {
            n232 = Build Array (concatenate)(w931, w930) -> (w929:dbl[][])
            n233 = Index Array(array=w930, index=0) -> (element=w928:dbl)
            n234 = Index Array(array=w930, index=1) -> (element=w927:dbl)
            n235 = disable-structure shown="Disabled" {
              disable-tunnel: w928 -> [w951 _]
              disable-tunnel: w927 -> [w950 _]
              disable-tunnel: w926 -> [w948 _]
              disable-tunnel: [w947 _] -> w925
              frame Disabled {
                # "DCS points DB stuff"
                n236 = Get Date/Time In Seconds() -> (seconds since 1Jan1904=w949:timestamp)
                n237 = call <userlib>:"timestamp_conversion.vi"("error in (no error)"=w948, "Time Stamp"=w949) -> ("error out"=w943:errorcluster, "Integer Time"=w946:i64)  [unwired: 7 in]
                n238 = Bundle By Name(cluster=T4 {"Integer Timestamp"=8, "X"=2.0, "Y"=3.0, "DCS spot ID"=0} ("DCS points"), "Integer Timestamp"=w946, "X"=w951, "Y"=w950) -> (w945:T4)
                n239 = call <userlib>:"post_dcs_points.vi"("error in (no error)"=w943, "DCS points"=w945) -> ("error out"=w947:errorcluster)  [unwired: 8 in, 1 out]
              }
              frame Enabled {
              }
            }
            n240 = Search 1D Array(1D array=w934, element=w928) -> (index of element=w939:i32)  [unwired: 1 in]
            n241 = Search 1D Array(1D array=w934, element=w927) -> (index of element=w938:i32)  [unwired: 1 in]
            n242 = Index Array(array=w940, index (row)=w939, index (col)=w938) -> (element=w937:dbl)
            n243 = Increment(x=w933) -> (x+1=w932:i32)
            n244 = Increment(x=w937) -> (x+1=w936:dbl)
            n245 = Replace Array Subset(array=w940, new element=w936, index (row)=w939, index (col)=w938) -> (w935:dbl[][])
          }
          frame True {
          }
        }
        n246 = local read "Tab Control"() -> (w290:T1)
        n247 = Equal?(x=w290, y=T1."DCS") -> (x = y?=w288:bool)
        n248 = case shown="True" w288 {
          tunnel: w298 -> [_ w713]
          frame False {
          }
          frame True {
            n249 = Array Max & Min(array=w713) -> (max value=w712:dbl)  [unwired: 3 out]
            n250 = Index Array(array="Color bar Control") -> (element=w721:cluster{dbl, u32})  [unwired: 1 in]
            n251 = Bundle(cluster=w721, 0.0, u32 0) -> (w722:cluster{dbl, u32})
            n252 = Bundle(cluster=w721, w712, u32 16448250) -> (w719:cluster{dbl, u32})
            n253 = Bundle(cluster=w721, 1.0, u32 16860) -> (w720:cluster{dbl, u32})
            n254 = Build Array(w722, w720, w719) -> (w711:cluster{dbl, u32}[])
            n255 = local write "Color bar Control"(w711) -> ()
            n256 = property on="Intensity Graph" class="IntGraph (strict)"("ZScale.MarkerVals[]"="Color bar Control") -> ()  [unwired: 2 in, 2 out]
            "Intensity Graph" <- w713
          }
        }
        n257 = Equal To 0?(x=w318) -> (x = 0?=w358:bool)
        n258 = local read "Particle Limit"() -> (w325:i64)
        n259 = Select(t=-1, s=w358, f=w318) -> (s? t:f=w324:i32)
        n260 = Quotient & Remainder(x=w297, y=10) -> (x-y*floor(x/y)=w346:i32)  [unwired: 1 out]
        n261 = Equal To 0?(x=w346) -> (x = 0?=w295:bool)
        n262 = Quotient & Remainder(x=w324, y=w325) -> (x-y*floor(x/y)=w356:i64)  [unwired: 1 out]
        n263 = Quotient & Remainder(x=w324, y="# of shots to calculate spot") -> (x-y*floor(x/y)=w323:i32)  [unwired: 1 out]
        n264 = case shown="True" w295 {
          tunnel: w347 -> [w841 w848]
          tunnel: [w841 w845] -> w333
          tunnel: [w840 w844] -> w332
          tunnel: w334 -> [w840 w843]
          tunnel: w318 -> [_ w844]
          frame False {
          }
          frame True {
            n265 = Get Date/Time In Seconds() -> (seconds since 1Jan1904=w849:timestamp)
            n266 = To Double Precision Float(number=w849) -> (double precision float=w845:dbl)
            n267 = Subtract(x=w845, y=w848) -> (x-y=w847:dbl)
            n268 = Subtract(x=w844, y=w843) -> (x-y=w842:i32)
            n269 = Divide(x=w842, y=w847) -> (x/y=→"Avg. Freq. (Hz)":dbl)
          }
        }
        n270 = Equal To 0?(x=w323) -> (x = 0?=w313:bool)
        n271 = Subtract(x=w325, y=w356) -> (x-y=→"Countdown to\nnext track point":i64)
        n272 = Equal To 0?(x=w356) -> (x = 0?=w314:bool)
        n273 = event shown="[2] \"Clear Spot/Track\": Value Change" {
          selector: _ -> [_ _ _]
          dyn-events: _ -> [_ _ _]
          timeout: 0 -> [_ _ _]
          tunnel: w327 -> [w781 w809 _]
          tunnel: w298 -> [w780 w810 _]
          tunnel: [w779 w808 w836] -> w336
          tunnel: w330 -> [w773 w800 _]
          tunnel: [w778 w807 dbl[][] []] -> w351
          tunnel: w318 -> [w771 w799 _]
          tunnel: [w771 w799 0] -> w317
          event Timeout {
            n274 = event-data() -> ()  [unwired: 1 in, 2 out]
            n275 = local read "Particle Limit"() -> (w774:i64)
            n276 = Array Size(array=w773) -> (size(s)=w777:i32[])
            n277 = Index Array(array=w777, index=0) -> (element=w775:i32)
            n278 = Greater?(x=w775, y=w774) -> (0:w772:bool)
            n279 = case shown="True" w772 {
              tunnel: w781 -> [_ w794]
              tunnel: w780 -> [w783 w789]
              tunnel: [w783 w788] -> w779
              tunnel: w773 -> [w782 w787]
              tunnel: [w782 w784] -> w778
              frame False {
              }
              frame True {
                n280 = Delete From Array(array=w787, index (row)=0) -> (deleted portion=w785:dbl[], array with subset deleted=w784:dbl[][])  [unwired: 2 in]
                n281 = Index Array(array=w785, index=0) -> (element=w795:dbl)
                n282 = Index Array(array=w785, index=1) -> (element=w796:dbl)
                n283 = Search 1D Array(1D array=w794, element=w795) -> (index of element=w790:i32)  [unwired: 1 in]
                n284 = Search 1D Array(1D array=w794, element=w796) -> (index of element=w791:i32)  [unwired: 1 in]
                n285 = Index Array(array=w789, index (row)=w790, index (col)=w791) -> (element=w793:dbl)
                n286 = Decrement(x=w793) -> (x-1=w792:dbl)
                n287 = Replace Array Subset(array=w789, new element=w792, index (row)=w790, index (col)=w791) -> (w788:dbl[][])
              }
            }
          }
          event "Particle Limit": Value Change {
            n288 = event-data() -> ()  [unwired: 1 in, 2 out]
            n289 = Array Size(array=w800) -> (size(s)=w806:i32[])
            n290 = Index Array(array=w806, index=0) -> (element=w804:i32)
            n291 = Greater?(x=w804, y="Particle Limit") -> (0:w801:bool)
            n292 = Subtract(x=w804, y="Particle Limit") -> (x-y=w802:i64)
            n293 = case shown="True" w801 {
              tunnel: w810 -> [w812 w816]
              tunnel: w800 -> [w811 w818]
              tunnel: w809 -> [_ w817]
              tunnel: [w811 w815] -> w807
              tunnel: [w812 w814] -> w808
              tunnel: w802 -> [_ w813]
              frame False {
              }
              frame True {
                n294 = for {
                  N: w813 -> [_]
                  tunnel: w817 -> [w823]
                  shift-right: [w819] -> w814
                  shift-left: w816 -> [w822]
                  shift-right: [w820] -> w815
                  shift-left: w818 -> [w824]
                  n295 = Delete From Array(array=w824, index (row)=0) -> (deleted portion=w821:dbl[], array with subset deleted=w820:dbl[][])  [unwired: 2 in]
                  n296 = Index Array(array=w821, index=0) -> (element=w830:dbl)
                  n297 = Index Array(array=w821, index=1) -> (element=w831:dbl)
                  n298 = Search 1D Array(1D array=w823, element=w830) -> (index of element=w826:i32)  [unwired: 1 in]
                  n299 = Search 1D Array(1D array=w823, element=w831) -> (index of element=w827:i32)  [unwired: 1 in]
                  n300 = Index Array(array=w822, index (row)=w826, index (col)=w827) -> (element=w829:dbl)
                  n301 = Decrement(x=w829) -> (x-1=w828:dbl)
                  n302 = Replace Array Subset(array=w822, new element=w828, index (row)=w826, index (col)=w827) -> (w819:dbl[][])
                }
              }
            }
          }
          event "Clear Spot/Track": Value Change {
            w837 = 49 ("dimension size")
            n303 = event-data() -> ()  [unwired: 1 in, 2 out]
            n304 = local write "Clear Spot/Track"(FALSE ("Clear Spot/Track")) -> ()
            n305 = Initialize Array(0.0 ("element"), w837, w837) -> (w836:dbl[][])
          }
        }
        n306 = case shown="True" "Save Spot Image" {
          tunnel: w320 -> [w755 w765]
          tunnel: [w755 w764] -> w319
          frame False {
          }
          frame True {
            n307 = local write "Save Spot Image"(FALSE ("Save Spot Image")) -> ()
            n308 = Format Into String(format string="%03d", initial string="Image", w765) -> (resulting string=w761:string)  [unwired: 1 in, 1 out]
            n309 = Concatenate Strings(w761, ".png" ("string")) -> (w762:string)
            n310 = Build Path(base path="Spot Save Folder", name or relative path=w762) -> (appended path=w763:path)
            n311 = invoke on="Intensity Graph" class="IntGraph (strict)" method="Get Image"("image depth"=32 ("Image Depth")) -> ("image data"=w759:T5)  [unwired: 5 in, 5 out]
            n312 = call <vilib>:"Check if File or Folder Exists.vi"("path"="Spot Save Folder") -> ("file or folder exists?"=w756:bool)  [unwired: 8 in, 2 out]
            n313 = Increment(x=w765) -> (x+1=w764:i32)
            n314 = case shown="True" w756 {
              tunnel: w763 -> [_ w770]
              tunnel: w759 -> [_ w769]
              frame False {
              }
              frame True {
                n315 = call <vilib>:"Write PNG File.vi"("image data"=w769, "path to PNG file"=w770) -> ()  [unwired: 8 in, 2 out]
              }
            }
          }
        }
        n316 = for {
          tunnel: w336 -> [w919] mode=indexing
          tunnel: [w917] -> w374 mode=indexing
          tunnel: [w916] -> w373 mode=indexing
          i -> [w918]
          n317 = for {
            tunnel: w919 -> [w921] mode=indexing
            tunnel: w918 -> [w924]
            tunnel: [w922] -> w916 mode=indexing
            tunnel: [w920] -> w917 mode=indexing
            i -> [w923]
            n318 = Multiply(x=w921, y=w924) -> (x*y=w920:dbl)
            n319 = Multiply(x=w921, y=w923) -> (x*y=w922:dbl)
          }
        }
        n320 = Add Array Elements(numeric array=w336) -> (sum=w339:dbl)
        "# of Particles\nin Spot" <- w339
        n321 = Add Array Elements(numeric array=w374) -> (sum=w372:dbl)
        n322 = Add Array Elements(numeric array=w373) -> (sum=w371:dbl)
        n323 = Divide(x=w372, y=w339) -> (x/y=w370:dbl)
        n324 = Divide(x=w371, y=w339) -> (x/y=w369:dbl)
        n325 = Subtract(x=w370, y=24.0) -> (x-y=w363:dbl)
        n326 = Subtract(x=w369, y=24.0) -> (x-y=w367:dbl)
        n327 = Divide(x=w363, y=2.0) -> (x/y=w301:dbl)
        n328 = Divide(x=w367, y=2.0) -> (x/y=w300:dbl)
        n329 = property on="Intensity Graph" class="IntGraph (strict)"(error in=w303, "Active Cursor"=u32 0, "Cursor.Cursor X"=w301, "Cursor.Cursor Y"=w300) -> (error out=w302:errorcluster)  [unwired: 1 in, 1 out]
        n330 = disable-structure shown="Disabled" {
          disable-tunnel: w364 -> [w381 _]
          disable-tunnel: [w380 _] -> w335
          disable-tunnel: [w379 _] -> w331
          disable-tunnel: "Load old position\nto Orange Cursor" -> [w378 _]
          disable-tunnel: w281 -> [w377 _]
          frame Disabled {
            n331 = case shown="True" w378 {
              tunnel: [w383 w388] -> w380
              tunnel: w381 -> [w383 w385]
              tunnel: w377 -> [w382 w390]
              tunnel: [w382 w389] -> w379
              frame False {
              }
              frame True {
                # "DCS DB loading stuff"
                n332 = call <userlib>:"querey dcs spot.vi"("error in (no error)"=w390) -> ("Spot"=w384:T3, "Cancel loading"=w387:bool, "error out"=w389:errorcluster)  [unwired: 15 in, 1 out]
                n333 = Unbundle By Name(w384) -> ("Spot X"=w392:dbl, "Spot Y"=w391:dbl)
                n334 = Build Array(w392, w391) -> (w386:dbl[])
                n335 = Select(t=w385, s=w387, f=w386) -> (s? t:f=w388:dbl[])
              }
            }
          }
          frame Enabled {
          }
        }
        n336 = Build Array(w301, w300) -> (w350:dbl[])
        "Current Spot Pos" <- w350
        n337 = case shown="True" w313 {
          tunnel: w352 -> [w852 w884]
          tunnel: [w852 w854] -> w349
          tunnel: w298 -> [_ w865]
          tunnel: w340 -> [w851 w864]
          tunnel: w350 -> [_ w862]
          tunnel: [w851 w863] -> w348
          tunnel: w339 -> [_ w858]
          tunnel: [w850 w857] -> w338
          tunnel: w303 -> [w850 w855]
          tunnel: w314 -> [_ w853]
          frame False {
          }
          frame True {
            w875 = sgl 0.0 ("element")
            w876 = sgl 2.0 ("element")
            # "DCS Spots DB stuff"
            n338 = Build Array (concatenate)(w864, w862) -> (w863:dbl[][])
            n339 = Array Max & Min(array=w865) -> (max value=w878:dbl, max index (indices)=w877:i32[])  [unwired: 2 out]
            n340 = Array Size(array=w865) -> (size(s)=w881:i32[])
            n341 = Index Array(array=w862) -> (element #1=w861:dbl, element #2=w860:dbl)  [unwired: 2 in]
            n342 = Multiply Array Elements(1:w881) -> (0:w882:i32)
            n343 = To Variant(anything=w881) -> (Variant=w880:variant)
            n344 = Build Array (concatenate)(w878, w877, w876, w876, w875, w875) -> (w874:dbl[])
            n345 = Reshape Array(w865, w882) -> (w879:dbl[])
            n346 = vi-ref <userlib>:"2DGaussianRotationModelwithOffset.vi"() -> (w883:refnum<vi>)
            n347 = call-poly <vilib>:"Nonlinear Curve Fit.vi"("Y"=w879, "f(x,a)"=w883, "data"=w880, "initial parameters"=w874, "error in (no error)"=w855, "termination"=cluster{"max iteration":i32, "tolerance":dbl} {"max iteration"=1000, "tolerance"=1e-08}) -> ("best fit parameters"=w867:dbl[], "error out"=w856:errorcluster)  [unwired: 4 in, 4 out]
            n348 = Array Subset(array=w867, index=3, length=2) -> (w870:dbl[])
            n349 = Divide(x=24.0 ("y"), y=49.0) -> (x/y=w866:dbl)
            n350 = Multiply(x=w870, y=w866) -> (x*y=w859:dbl[])
            n351 = flat-sequence {
              tunnel: w884 -> [w895]
              tunnel: w861 -> [w894]
              tunnel: w860 -> [w893]
              tunnel: w859 -> [w892]
              tunnel: w858 -> [w889]
              tunnel: [w888] -> w857
              tunnel: w856 -> [w887]
              tunnel: [w886] -> w854
              tunnel: w853 -> [w885]
              frame #0 {
                n352 = Build Array (concatenate)(w895, w892) -> (w886:dbl[][])
                n353 = Index Array(array=w892) -> (element #1=w891:dbl, element #2=w890:dbl)  [unwired: 2 in]
                n354 = case shown="True" w885 {
                  tunnel: w894 -> [_ w903]
                  tunnel: w893 -> [_ w902]
                  tunnel: w891 -> [_ w901]
                  tunnel: w890 -> [_ w900]
                  tunnel: w889 -> [_ w899]
                  tunnel: [w896 w898] -> w888
                  tunnel: w887 -> [w896 w897]
                  frame False {
                  }
                  frame True {
                    n355 = disable-structure shown="Disabled" {
                      disable-tunnel: w903 -> [w911 _]
                      disable-tunnel: w902 -> [w910 _]
                      disable-tunnel: w901 -> [w909 _]
                      disable-tunnel: w900 -> [w908 _]
                      disable-tunnel: w899 -> [w907 _]
                      disable-tunnel: [w905 _] -> w898
                      disable-tunnel: w897 -> [w904 _]
                      frame Disabled {
                        n356 = Get Date/Time In Seconds() -> (seconds since 1Jan1904=w912:timestamp)
                        n357 = call <userlib>:"timestamp_conversion.vi"("error in (no error)"=w904, "Time Stamp"=w912) -> ("error out"=w906:errorcluster, "Integer Time"=w915:i64)  [unwired: 7 in]
                        n358 = Bundle By Name(cluster=T3 {"DCS spot ID"=0, "Integer Timestamp"=2, "Spot X"=3.0, "Spot Y"=4.0, "Spot Width X"=0.0, "Spot Width Y"=0.0, "Spot Size"=0, "Experiment Settings ID"=0} ("dcs_spot"), "Integer Timestamp"=w915, "Spot X"=w911, "Spot Y"=w910, "Spot Width X"=w909, "Spot Width Y"=w908, "Spot Size"=w907) -> (w914:T3)
                        n359 = call <userlib>:"post_dcs_spot.vi"("error in (no error)"=w906, "dcs_spot"=w914) -> ("error out"=w905:errorcluster)  [unwired: 8 in, 1 out]
                      }
                      frame Enabled {
                      }
                    }
                  }
                }
                "Spot Widths" <- w892
              }
            }
          }
        }
        n360 = Subtract(x="Orange Cursor Position", y=w350) -> (x-y=w345:dbl[])
        n361 = Multiply(x=w345, y=8.6106) -> (x*y=w343:dbl[])
        n362 = Select(t=w335, s="Load old position\nto Orange Cursor", f=w350) -> (s? t:f=w307:dbl[])
        n363 = Or(x="Load old position\nto Orange Cursor", y="Set Orange Cursor\nto current position") -> (x .or. y?=w306:bool)
        n364 = Divide(x=w343, y=2.0) -> (x/y=→"Laser spot\nMove (mm)":dbl[])
        n365 = case shown="True" w306 {
          tunnel: "Orange Cursor Position" -> [w742 _]
          tunnel: w307 -> [_ w749]
          tunnel: 1 -> [w739 w747]
          tunnel: w302 -> [w738 w744]
          tunnel: [w737 w743] -> w304
          frame False {
            n366 = Index Array(array=w742) -> (element #1=w741:dbl, element #2=w740:dbl)  [unwired: 2 in]
            n367 = property on="Intensity Graph" class="IntGraph (strict)"(error in=w738, "Active Cursor"=w739, "Cursor.Cursor X"=w741, "Cursor.Cursor Y"=w740) -> (error out=w737:errorcluster)  [unwired: 1 in, 1 out]
          }
          frame True {
            n368 = Index Array(array=w749) -> (element #1=w746:dbl, element #2=w745:dbl)  [unwired: 2 in]
            n369 = local write "Set Orange Cursor\nto current position"(FALSE ("Set Orange Cursor\nto current position")) -> ()
            n370 = local write "Orange Cursor Position"(w749) -> ()
            n371 = property on="Intensity Graph" class="IntGraph (strict)"(error in=w744, "Active Cursor"=w747, "Cursor.Cursor X"=w746, "Cursor.Cursor Y"=w745) -> (error out=w743:errorcluster)  [unwired: 1 in, 1 out]
          }
        }
        n372 = local read "Tab Control"() -> (w292:T1)
        n373 = local read "Tab Control"() -> (w312:T1)
        n374 = Equal?(x=w292, y=T1."DCS") -> (x = y?=w291:bool)
        n375 = Equal?(x=w312, y=T1."Spot Size Tracking") -> (x = y?=w294:bool)
        n376 = case shown="True" w291 {
          tunnel: w348 -> [_ w734]
          tunnel: w338 -> [w724 w733]
          tunnel: [w724 w732] -> w337
          frame False {
          }
          frame True {
            n377 = Index Array(array=w734, index (col)=0 ("disabled index (col)")) -> (element=w728:dbl[])  [unwired: 1 in]
            n378 = Index Array(array=w734, index (col)=1 ("disabled index (col)")) -> (element=w726:dbl[])  [unwired: 1 in]
            n379 = call "Convert to Dynamic Data"("Array"=w728) -> ("Dynamic Data Type"=w727:dynamicdata)  [unwired: 3 in]
            n380 = call "Convert to Dynamic Data2"("Array"=w726) -> ("Dynamic Data Type"=w725:dynamicdata)  [unwired: 3 in]
            n381 = call "Build XY Graph"("error in (no error)"=w733, "Y Input"=w725, "X Input"=w727) -> ("error out"=w732:errorcluster, "XY Graph"=→"XY Graph":cluster{"Y":dbl[], "Y":dbl[]}[])  [unwired: 2 in, 5 out]
          }
        }
        n382 = case shown="True" w294 {
          tunnel: w349 -> [_ w736]
          frame False {
          }
          frame True {
            n383 = Transpose 2D Array(2D array=w736) -> (transposed array=→"Spot Size over time":dbl[][])
          }
        }
        n384 = Merge Errors(w337, w304, w331) -> (w326:errorcluster)
        "Running Errors" <- w281
      }
      n385 = Not(x=w46) -> (.not. x?=w40:bool)
      n386 = Not Equal To 0?(x=w41) -> (x != 0?=w39:bool)
      n387 = disable-structure shown="Disabled" {
        disable-tunnel: w54 -> [w82 _]
        disable-tunnel: w45 -> [w81 _]
        disable-tunnel: w40 -> [w80 _]
        disable-tunnel: w39 -> [w78 _]
        frame Disabled {
          n388 = And(x=w78, y=w80) -> (x .and. y?=w79:bool)
          n389 = case shown="True" w79 {
            tunnel: w82 -> [_ w93]
            tunnel: w81 -> [_ w89]
            frame False {
            }
            frame True {
              # "Stuff to post last spot on shutdown"
              n390 = Index Array(array=w93) -> (element #1=w92:dbl, element #2=w91:dbl)  [unwired: 2 in]
              n391 = Array Size(array=w89) -> (size(s)=w90:i32[])
              n392 = local read "# of Particles\nin Spot"() -> (w83:dbl)
              n393 = Get Date/Time In Seconds() -> (seconds since 1Jan1904=w97:timestamp)
              n394 = Index Array(array=w90) -> (element=w88:i32)  [unwired: 1 in]
              n395 = call <userlib>:"timestamp_conversion.vi"("Time Stamp"=w97) -> ("Integer Time"=w96:i64)  [unwired: 8 in, 1 out]
              n396 = Index Array(array=w89, index (row) #1=w88, index (col) #1=0 ("disabled index (col)"), index (row) #2=w88, index (col) #2=1 ("disabled index (col)")) -> (element #1=w87:dbl, element #2=w84:dbl)
              n397 = Bundle By Name(cluster=T3 {"DCS spot ID"=0, "Integer Timestamp"=2, "Spot X"=3.0, "Spot Y"=4.0, "Spot Width X"=0.0, "Spot Width Y"=0.0, "Spot Size"=0, "Experiment Settings ID"=0} ("dcs_spot"), "Integer Timestamp"=w96, "Spot X"=w92, "Spot Y"=w91, "Spot Width X"=w87, "Spot Width Y"=w84, "Spot Size"=w83) -> (w94:T3)
              n398 = call <userlib>:"post_dcs_spot.vi"("dcs_spot"=w94) -> ()  [unwired: 9 in, 2 out]
            }
          }
        }
        frame Enabled {
        }
      }
    }
    frame Error {
    }
  }
  "error out" <- w13
